vi "Actor Core.vi"(8 "error in":errorcluster, 11 "Transfer Line in":refnum<class "Transfer Line.lvclass">) -> (0 "error out":errorcluster, 3 "Actor out":refnum<class "Actor.lvclass">)   [LabVIEW 2015, in "cRIO-Carbondioxide.lvlib" / "CO2-Actor.lvlib" / "Transfer Line.lvclass"]
doc: "(<B>Filename</B>: Actor Framework.lvlib:Actor.lvclass:Actor Core.vi)\n\nReceives messages to the actor, reacts to them, and initiates any error handling that may shut the actor down.\n\nDescendant classes may override this VI to append parallel tasks for the actor to complete while it handles messages. Overrides use the Call Parent Method node."
uses:
  Transfer Line.lvclass
  <vilib>/ActorFramework/Actor/Actor.lvclass
  CO2 Actor/CO2 Actor.lvclass
  Transfer Line.lvclass/Transfer Line.ctl
  subs/Sample/Read Sample From Container.vi
  subs/Sample/Sample.lvclass
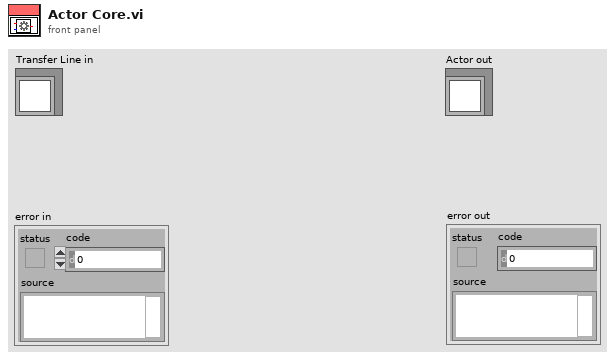
[diagram p1: front panel]
types:
  T1 = typedef "Sample Container.ctl" = cluster{"Sample In":refnum<k21>, "Sample Name":refnum<k21>, "Ti Cathode":refnum<k21>, "SampleQ":refnum<queue>}
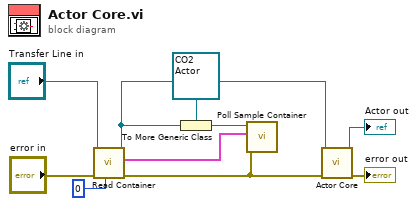
[diagram p0: block diagram]
diagram:
  n1 = call "Read Container.vi"("Queue timeout in ms (-1)"=0, "error in (no error)"="error in", "Transfer Line in"="Transfer Line in") -> ("error out"=w7:errorcluster, "Sample Container"=w2:T1, "Transfer Line out"=w5:refnum<class "Transfer Line.lvclass">)  [unwired: 4 in, 2 out]
  n2 = To More Generic Class(target class=refnum<class "CO2 Actor.lvclass"> refnum ("CO2 Actor in"), reference=w5) -> (generic class reference=w3:refnum<class "CO2 Actor.lvclass">)
  n3 = call-dynamic "Poll Sample Container.vi"("error in (no error)"=w7, "Sample Container"=w2, "CO2 Actor in"=w3) -> ()  [unwired: 8 in, 1 out]
  n4 = call-parent "Actor Core.vi"("error in"=w7, "CO2 Actor in"=w5) -> ("error out"=→"error out":errorcluster, "Actor out"=→"Actor out":refnum<class "Actor.lvclass">)  [unwired: 8 in]
